vi "Control Relay (boolean).vi"(8 "error in (no error)":errorcluster, 9 "Array":bool[](array[boolean])) -> (0 "error out":errorcluster)   [LabVIEW 2019, in "Relay-Box.lvclass"]
uses:
  Relay-Box.lvclass
  Relay-Box.lvclass/Relay-Box.ctl
  <instrlib>/FTDI/D2XX/D2XX.lvlib
panel:
  out "FT_Status out":u32(ring) items=["FT_OK", "FT_INVALID_HANDLE", "FT_DEVICE_NOT_FOUND", "FT_DEVICE_NOT_OPENED", "FT_IO_ERROR", "FT_INSUFFICIENT_RESOURCES", "FT_INVALID_PARAMETER", "FT_INVALID_BAUD_RATE", "FT_DEVICE_NOT_OPENED_FOR_ERASE", "FT_DEVICE_NOT_OPENED_FOR_WRITE", "FT_FAILED_TO_WRITE_DEVICE", "FT_EEPROM_READ_FAILED", "FT_EEPROM_WRITE_FAILED", "FT_EEPROM_ERASE_FAILED", "FT_EEPROM_NOT_PRESENT", "FT_EEPROM_NOT_PROGRAMMED", "FT_INVALID_ARGS", "FT_NOT_SUPPORTED", "FT_OTHER_ERROR"]
  # "Discharge tip"
  # "0 ohm"
  # "100k ohm"
  # "10M ohm"
  # "1Gohm"
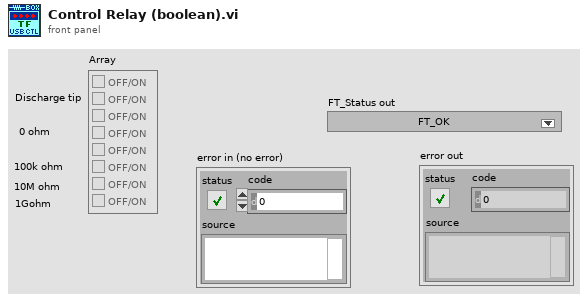
[diagram p1: front panel]
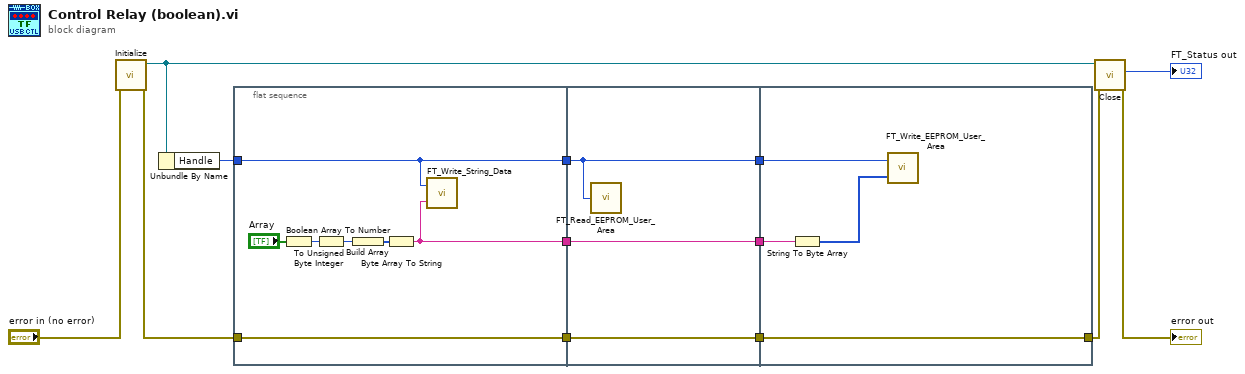
[diagram p0: block diagram]
diagram:
  n1 = call "Initialize.vi"("error in (no error)"="error in (no error)") -> ("error out"=w6:errorcluster, "Relay-Box out"=w5:refnum<class "Relay-Box.lvclass">)  [unwired: 9 in]
  n2 = Unbundle By Name(w5) -> ("Handle"=w2:u32)
  n3 = flat-sequence {
    tunnel: [w15] -> w13
    tunnel: [w20] -> w12
    tunnel: [w14] -> w11
    tunnel: w6 -> [w20]
    tunnel: w2 -> [w15]
    tunnel: w13 -> [w22]
    tunnel: [w22] -> w10
    tunnel: w12 -> [w23]
    tunnel: [w23] -> w9
    tunnel: w11 -> [w21]
    tunnel: [w21] -> w1
    tunnel: w10 -> [w26]
    tunnel: w9 -> [w27]
    tunnel: [w27] -> w3
    tunnel: w1 -> [w25]
    frame #0 {
      n4 = Boolean Array To Number(Boolean array="Array") -> (number=w17:u32)
      n5 = To Unsigned Byte Integer(number=w17) -> (unsigned 8bit integer=w19:u8)
      n6 = Build Array(w19) -> (w18:u8[])
      n7 = Byte Array To String(unsigned byte array=w18) -> (string=w14:string)
      n8 = call <instrlib>:"FT_Write_String_Data.vi"("Buffer"=w14, "Handle"=w15) -> ()  [unwired: 2 out]
    }
    frame #1 {
      n9 = call <instrlib>:"FT_Read_EEPROM_User_Area.vi"("Handle"=w22) -> ()  [unwired: 3 out]
    }
    frame #2 {
      n10 = String To Byte Array(string=w25) -> (unsigned byte array=w24:u8[])
      n11 = call <instrlib>:"FT_Write_EEPROM_User_Area.vi"("User Area Data In"=w24, "Handle"=w26) -> ()  [unwired: 1 out]
    }
  }
  n12 = call "Close.vi"("error in (no error)"=w3, "Relay-Box in"=w5) -> ("error out"=→"error out":errorcluster, "FT_Status"=→"FT_Status out":u32)  [unwired: 7 in, 1 out]
